vi "LVClass_HasoEngine Set Preferences.vi"(0 "HasoEngine in":refnum<class "HasoEngine.lvclass">, 5 "Slopes_HasoEngine_Setup":T1={"Start sub-aperture"={"X"=85, "Y"=63}, "Pupil average"=670.0, "AutoStartSub-aperture"=FALSE} {"Pupil average" min=0.0 max=1.0}, 11 "error in (no error)":errorcluster) -> (4 "HasoEngine out":refnum<class "HasoEngine.lvclass">, 15 "error out":errorcluster)   [LabVIEW 2020, in "HasoEngine.lvclass"]
doc: "HasoSlopes computation preferences setter.\n\n--------------------------------------------------------------------------------\n\n<B>HasoEngineIn </B> : HasoEngine object.\n<B>HasoEngineOut </B> : HasoEngine object.\n<B>start_subpupil </B> : Coordinates of the first calculated sub-pupil (index coordinates relative to\n the top-left corner of the pupil).\n<B>denoising_strength </B> : Sensitivity of spot detection on summed images (between 0 and 1).\n<B>ErrorIn </B> : Error\n<B>ErrorOut </B> : Error\n\n--------------------------------------------------------------------------------"
uses:
  HasoEngine.lvclass
  SlopesEngineSetup.ctl
  Point2D.ctl
  HasoEngine.lvclass/HasoEngine.ctl
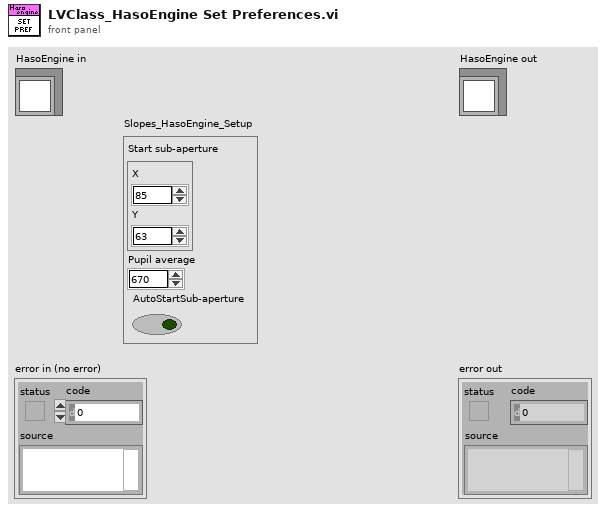
[diagram p1: front panel]
types:
  T1 = typedef "SlopesEngineSetup.ctl" = cluster{"Start sub-aperture":T2, "Pupil average":dbl, "AutoStartSub-aperture":bool}
  T2 = typedef "Point2D.ctl" = cluster{"X":u32, "Y":u32}
  T3 = typedef "ClassID.ctl" = i64
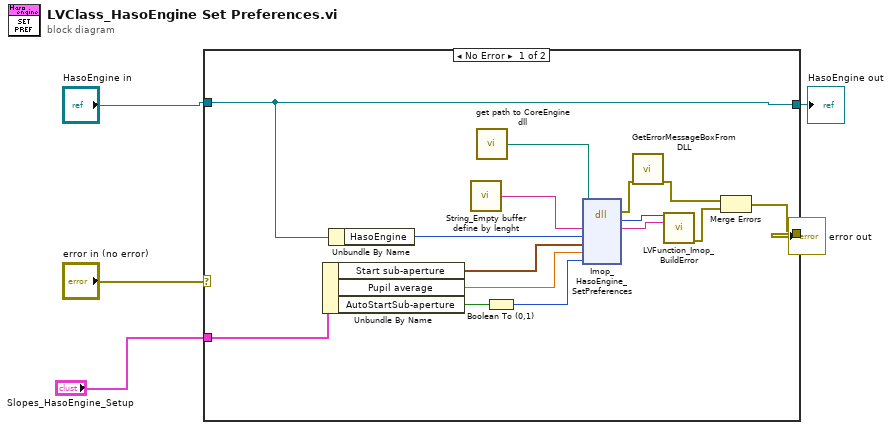
[diagram p0: block diagram]
diagram:
  n1 = case shown="No Error" "error in (no error)" {
    selector: "error in (no error)" -> [_ w21]
    tunnel: "HasoEngine in" -> [w12 w22]
    tunnel: [w12 w22] -> w2
    tunnel: [w8 w21] -> w3
    tunnel: "Slopes_HasoEngine_Setup" -> [w15 _]
    frame No Error {
      n2 = Unbundle By Name(w15) -> ("Start sub-aperture"=w14:T2, "Pupil average"=w13:dbl, "AutoStartSub-aperture"=w7:bool)
      n3 = Unbundle By Name(w12) -> ("HasoEngine"=w11:T3)
      n4 = call "String_Empty buffer define by lenght.vi"() -> ("Empty buffer"=w18:string)  [unwired: 1 in]
      n5 = call "get path to CoreEngine dll.vi"() -> ("path to wavekit library"=w17:path)  [unwired: 14 in, 1 out]
      n6 = Boolean To (0,1)(Boolean=w7) -> (0, 1=w6:i16)
      n7 = dll-call lib="D:/2_trunk/Soft_haso/ImOpCoreEngine4_LV2011/DLLs/ImopEngine4_vc100.dll" fn="Imop_HasoEngine_SetPreferences"(path in=w17, "message"=w18, "objet"=w11, "StartSubPupil"=w14, "pupil_average"=w13, "AutoStartSub-aperture"=w6) -> (error out=w16:errorcluster, "return type"=w19:i32, "message"=w20:string)  [unwired: 6 in, 1 out]
      n8 = call "GetErrorMessageBoxFromDLL.vi"("error IN"=w16) -> ("error OUT"=w10:errorcluster)  [unwired: 10 in]
      n9 = call "LVFunction_Imop_BuildError.vi"("code"=w19, "String to Prepend to source (\"\")"=w20) -> ("error out"=w9:errorcluster)  [unwired: 13 in]
      n10 = Merge Errors(w10, w9) -> (w8:errorcluster)
    }
    frame Error {
    }
  }
  "error out" <- w3
  "HasoEngine out" <- w2
